vi "sub vi - AI USB4704 (3) v72.vi"(0 "Task0":i32, 5 "Task1":i32, 7 "Task2":i32) -> (1 "Graph 1":waveform(dbl)[](graph), 2 "Graph 2":waveform(dbl)[](graph), 3 "Graph 3":waveform(dbl)[](graph), 10 "loop time":dbl format="%.6g", 15 "error array":errorcluster[](array[cluster]))   [LabVIEW 2017]
uses:
  program files/Global 1.vi
  <userlib>/DAQNavi Polymorphic VI/read/DAQNavi Read (Analog 1D Wfm NChan NSamp).vi
panel:
  in  "SAMPLES":dbl
  in  "Tab Control":enum32{"USB #0", "USB #1", "USB #2"}(tab)
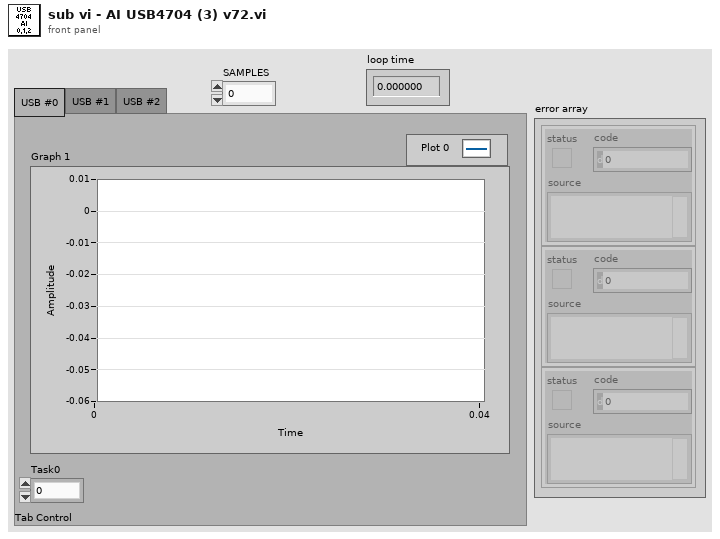
[diagram p1: front panel]
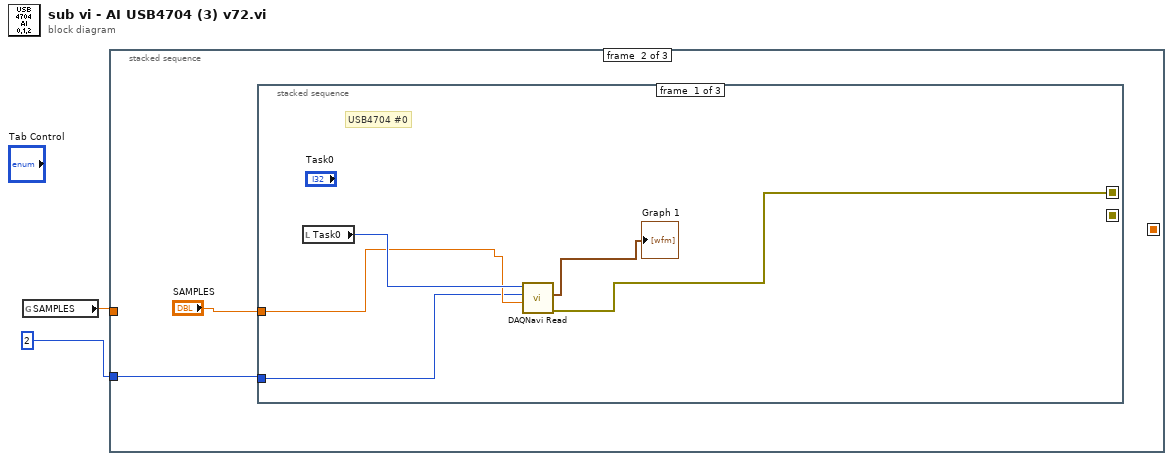
[diagram p0: block diagram]
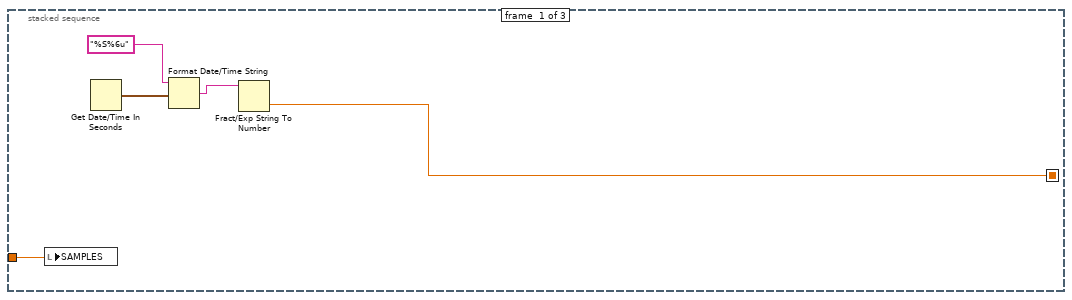
[diagram p2: hidden frame]
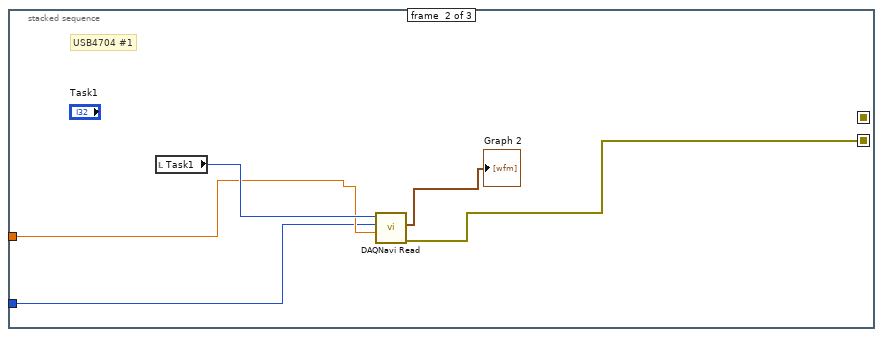
[diagram p3: hidden frame]
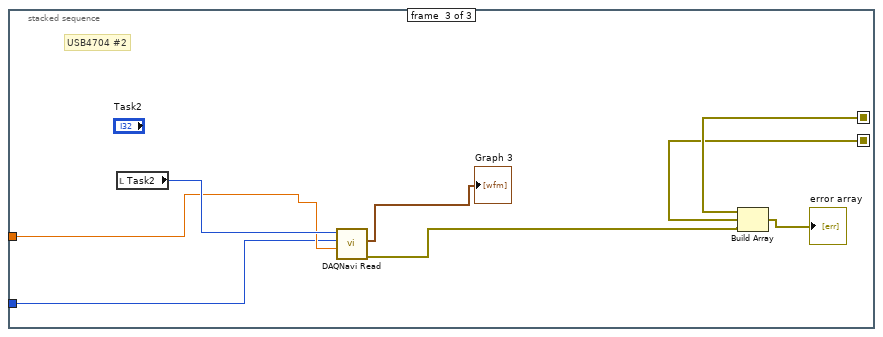
[diagram p4: hidden frame]
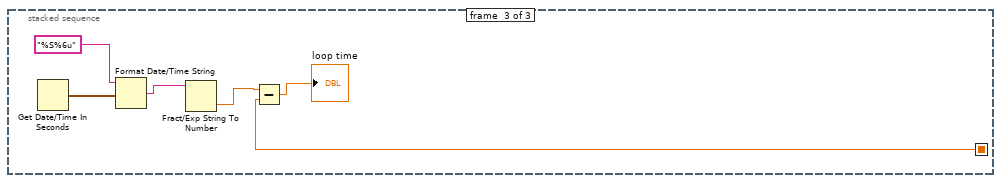
[diagram p5: hidden frame]
diagram:
  n1 = global read "Global 1.vi" "SAMPLES"() -> (w1:dbl)
  n2 = stacked-sequence {
    seq-local: [w4 _ _] -> [_ _ w29]
    tunnel: 2 -> [_ w9 _]
    tunnel: w1 -> [w3 _ _]
    frame #0 {
      n3 = local write "SAMPLES"(w3) -> ()
      n4 = Get Date/Time In Seconds() -> (seconds since 1Jan1904=w6:timestamp)
      n5 = Format Date/Time String(time format string (%c)="%S%6u", seconds (now)=w6) -> (date/time string=w5:string)  [unwired: 1 in]
      n6 = Fract/Exp String To Number(string=w5) -> (number=w4:dbl)  [unwired: 3 in, 1 out]
    }
    frame #1 {
      n7 = stacked-sequence {
        seq-local: [w11 _ _] -> [_ _ w23]
        seq-local: [_ w17 _] -> [_ _ w22]
        tunnel: "SAMPLES" -> [w13 w16 w26]
        tunnel: w9 -> [w10 w15 w20]
        frame #0 {
          # "USB4704 #0"
          n8 = local read "Task0"() -> (w14:i32)
          n9 = call-poly <userlib>:"DAQNavi Read.vi"("number of samples per channel to read"=w13, "timeout"=w10, "task in"=w14) -> ("error out"=w11:errorcluster, "data"=→"Graph 1":waveform(dbl)[])  [unwired: 1 in, 6 out]
        }
        frame #1 {
          # "USB4704 #1"
          n10 = local read "Task1"() -> (w19:i32)
          n11 = call-poly <userlib>:"DAQNavi Read.vi"("number of samples per channel to read"=w16, "timeout"=w15, "task in"=w19) -> ("error out"=w17:errorcluster, "data"=→"Graph 2":waveform(dbl)[])  [unwired: 1 in, 6 out]
        }
        frame #2 {
          # "USB4704 #2"
          n12 = local read "Task2"() -> (w27:i32)
          n13 = call-poly <userlib>:"DAQNavi Read.vi"("number of samples per channel to read"=w26, "timeout"=w20, "task in"=w27) -> ("error out"=w24:errorcluster, "data"=→"Graph 3":waveform(dbl)[])  [unwired: 1 in, 6 out]
          n14 = Build Array(w23, w22, w24) -> (→"error array":errorcluster[])
        }
      }
    }
    frame #2 {
      n15 = Get Date/Time In Seconds() -> (seconds since 1Jan1904=w32:timestamp)
      n16 = Format Date/Time String(time format string (%c)="%S%6u", seconds (now)=w32) -> (date/time string=w31:string)  [unwired: 1 in]
      n17 = Fract/Exp String To Number(string=w31) -> (number=w30:dbl)  [unwired: 3 in, 1 out]
      n18 = Subtract(x=w30, y=w29) -> (x-y=→"loop time":dbl)
    }
  }
